vi "WPI_DashboardProcessTCPPacket.vi"(11 "data in":string) -> (1 "New Robot IP":bool, 2 "Docked":bool, 3 "Robot IP":string, 4 "Power and Errors":T1, 5 "Simulated":bool)   [LabVIEW 2025]
uses:
  <vilib>/Utility/config.llb/Read Key (String).vi
  <vilib>/Utility/config.llb/Write Key (String).vi
  <vilib>/Utility/config.llb/NI_LVConfig.lvlib
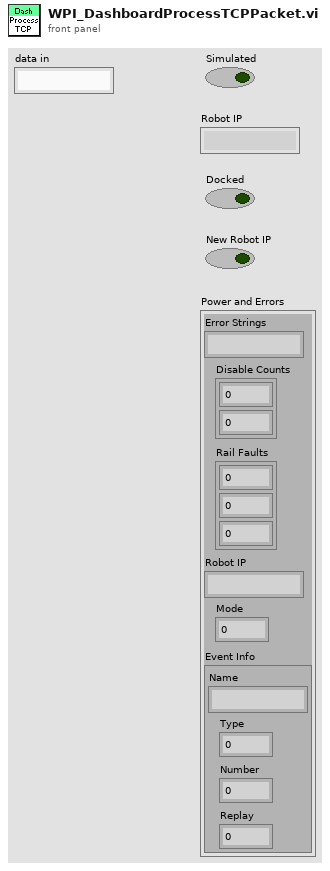
[diagram p1: front panel]
types:
  T1 = cluster{"Error Strings":string, "Disable Counts":cluster{u16, u16}, "Rail Faults":cluster{u16, u16, u16}, "Robot IP":string, "Mode":u8, "Event Info":cluster{"Name":string, "Type":u8, "Number":u16, "Replay":u8}}
  T2 = cluster{"Error Strings":string, "Disable Counts":cluster{u16, u16}, "Rail Faults":cluster{u16, u16, u16}, "Robot IP":string, "Mode":u8, "Event Info":cluster{"Name":string, "Type":u8, "Number":u16, "Replay":u8}, "New Robot IP":bool}
  T3 = typedef "NI_LVConfig.lvlib/Config Data RefNum.ctl" = refnum<k1>
  T4 = cluster{"Name":string, "Type":u8, "Number":u16, "Replay":u8}
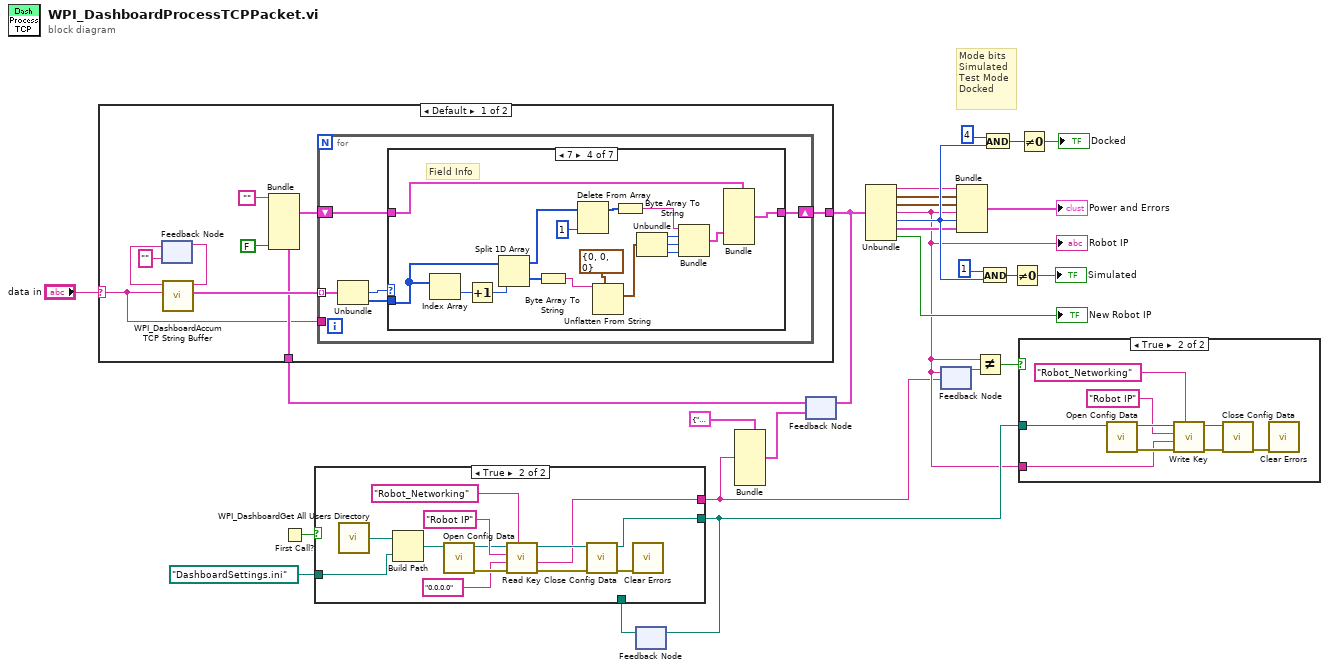
[diagram p0: block diagram]
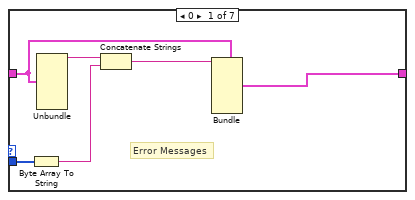
[diagram p4: hidden frame]
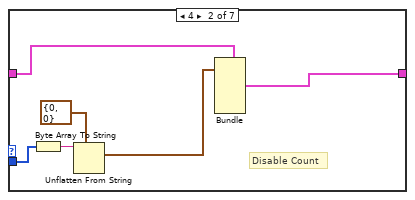
[diagram p5: hidden frame]
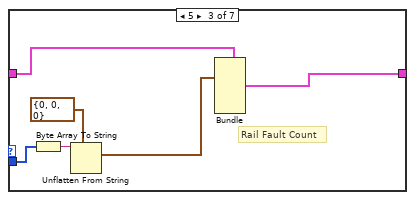
[diagram p6: hidden frame]
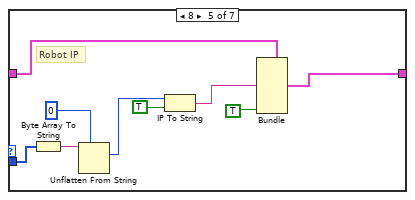
[diagram p7: hidden frame]
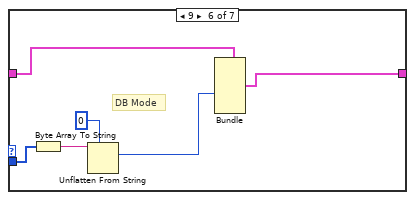
[diagram p8: hidden frame]
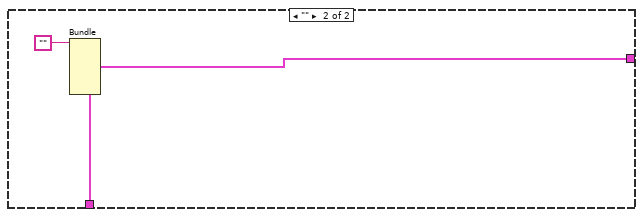
[diagram p10: hidden frame]
diagram:
  # "Mode bits\nSimulated\nTest Mode\nDocked"
  n1 = First Call?() -> (First Call?: T/F=w10:bool)
  n2 = feedback #1() -> (w3:path)  [unwired: 1 in]
  n3 = case shown="True" w10 {
    tunnel: path "DashboardSettings.ini" -> [_ w31]
    tunnel: [_ w29] -> w1
    tunnel: [w27 w28] -> w4
    tunnel: w3 -> [w27 _]
    frame False {
    }
    frame True {
      n4 = call <vilib>:"WPI_DashboardGet All Users Directory.vi"() -> ("All User Path"=w40:path)
      n5 = Build Path(base path=w40, name or relative path=w31) -> (appended path=w39:path)
      n6 = call <vilib>:"Open Config Data.vi"("configuration file path"=w39) -> ("error out"=w33:errorcluster, "refnum"=w36:T3)  [unwired: 8 in, 1 out]
      n7 = call-poly <vilib>:"Read Key.vi"("section"="Robot_Networking", "error in (no error)"=w33, "default value"="0.0.0.0", "key"="Robot IP", "refnum"=w36) -> ("error out"=w32:errorcluster, "value"=w29:string, "refnum out"=w34:T3)  [unwired: 1 in, 3 out]
      n8 = call <vilib>:"Close Config Data.vi"("error in (no error)"=w32, "refnum"=w34) -> ("error out"=w35:errorcluster, "file path"=w28:path)  [unwired: 1 in, 7 out]
      n9 = call <vilib>:"Clear Errors.vi"("error in (no error)"=w35) -> ()  [unwired: 5 in, 2 out]
    }
  }
  n10 = feedback-in #1(w4) -> ()
  n11 = Bundle(cluster=T2 {"Error Strings"="", "Disable Counts"={0, 0}, "Rail Faults"={0, 0, 0}, "Robot IP"="", "Mode"=0, "Event Info"={"Name"="", "Type"=0, "Number"=0, "Replay"=0}, "New Robot IP"=FALSE} ("Robot Info"), "Robot IP"=w1) -> (w7:T2)  [unwired: 6 in]
  n12 = feedback #2(w7) -> (w11:T2)
  n13 = case shown="Default" "data in" {
    selector: "data in" -> [w42 _]
    tunnel: [w46 w109] -> w18
    tunnel: w11 -> [w44 w108]
    frame Default {
      n14 = feedback #3("" ("string")) -> (w49:string)
      n15 = call <vilib>:"WPI_DashboardAccum TCP String Buffer.vi"("data in"=w42, "string in"=w49) -> ("Array"=w47:cluster{u16, u8, "unsigned byte array":u8[]}[], "string out"=w48:string)  [unwired: 8 in]
      n16 = feedback-in #3(w48) -> ()
      n17 = Bundle(cluster=w44, "Error Strings"="", "New Robot IP"=FALSE) -> (w43:T2)  [unwired: 5 in]
      n18 = for {
        tunnel: w47 -> [w53] mode=indexing
        shift-right: [w51] -> w46
        shift-left: w43 -> [w52]
        tunnel: w42 -> [_]
        n19 = Unbundle(w53) -> (w55:u8, "unsigned byte array"=w54:u8[])  [unwired: 1 out]
        n20 = case shown="7" w55 {
          tunnel: w54 -> [w61 w67 w73 w86 w99 w105 _]
          tunnel: w52 -> [w60 w65 w71 w90 w98 w104 w106]
          tunnel: [w56 w64 w70 w89 w97 w103 w106] -> w51
          frame 0 {
            # "Error Messages"
            n21 = Byte Array To String(unsigned byte array=w61) -> (string=w58:string)
            n22 = Unbundle(w60) -> ("Error Strings"=w59:string)  [unwired: 6 out]
            n23 = Concatenate Strings(w59, w58) -> (w57:string)
            n24 = Bundle(cluster=w60, "Error Strings"=w57) -> (w56:T2)  [unwired: 6 in]
          }
          frame 4 {
            # "Disable Count"
            n25 = Byte Array To String(unsigned byte array=w67) -> (string=w66:string)
            n26 = Unflatten From String(type=cluster{u16, u16} {0, 0}, binary string=w66) -> (value=w62:cluster{u16, u16})  [unwired: 3 in, 2 out]
            n27 = Bundle(cluster=w65, "Disable Counts"=w62) -> (w64:T2)  [unwired: 6 in]
          }
          frame 5 {
            # "Rail Fault Count"
            n28 = Byte Array To String(unsigned byte array=w73) -> (string=w72:string)
            n29 = Unflatten From String(type=cluster{u16, u16, u16} {0, 0, 0}, binary string=w72) -> (value=w68:cluster{u16, u16, u16})  [unwired: 3 in, 2 out]
            n30 = Bundle(cluster=w71, "Rail Faults"=w68) -> (w70:T2)  [unwired: 6 in]
          }
          frame 7 {
            # "Field Info"
            n31 = Index Array(array=w86) -> (element=w88:u8)  [unwired: 1 in]
            n32 = Increment(x=w88) -> (x+1=w87:u8)
            n33 = Split 1D Array(array=w86, index=w87) -> (first subarray=w82:u8[], second subarray=w84:u8[])
            n34 = Byte Array To String(unsigned byte array=w84) -> (string=w83:string)
            n35 = Delete From Array(array=w82, index=1) -> (array with subset deleted=w80:u8[])  [unwired: 1 in, 1 out]
            n36 = Unflatten From String(type=cluster{u8, u16, u8} {0, 0, 0}, binary string=w83) -> (value=w77:cluster{u8, u16, u8})  [unwired: 3 in, 2 out]
            n37 = Byte Array To String(unsigned byte array=w80) -> (string=w79:string)
            n38 = Unbundle(w77) -> (w76:u8, w75:u16, w74:u8)
            n39 = Bundle("string"=w79, w76, w75, w74) -> (w78:cluster{"string":string, u8, u16, u8})  [unwired: 1 in]
            n40 = Bundle(cluster=w90, "Event Info"=w78) -> (w89:T2)  [unwired: 6 in]
          }
          frame 8 {
            # "Robot IP"
            n41 = Byte Array To String(unsigned byte array=w99) -> (string=w96:string)
            n42 = Unflatten From String(type=u32 0, binary string=w96) -> (value=w92:u32)  [unwired: 3 in, 2 out]
            n43 = IP To String(1:TRUE ("dot notation? (F)"), 2:w92) -> (0:w91:string)
            n44 = Bundle(cluster=w98, "Robot IP"=w91, "New Robot IP"=TRUE) -> (w97:T2)  [unwired: 5 in]
          }
          frame 9 {
            # "DB Mode"
            n45 = Byte Array To String(unsigned byte array=w105) -> (string=w101:string)
            n46 = Unflatten From String(type=u8 0, binary string=w101) -> (value=w100:u8)  [unwired: 3 in, 2 out]
            n47 = Bundle(cluster=w104, "Mode"=w100) -> (w103:T2)  [unwired: 6 in]
          }
          frame Default {
          }
        }
      }
    }
    frame "" {
      n48 = Bundle(cluster=w108, "Error Strings"="") -> (w109:T2)  [unwired: 6 in]
    }
  }
  n49 = feedback-in #2(w18) -> ()
  n50 = Unbundle(w18) -> ("Error Strings"=w13:string, "Disable Counts"=w16:cluster{u16, u16}, "Rail Faults"=w15:cluster{u16, u16, u16}, "Robot IP"=w2:string, "Mode"=w25:u8, "Event Info"=w14:T4, "New Robot IP"=→"New Robot IP":bool)
  "Robot IP" <- w2
  n51 = feedback #4(w1) -> (w6:string)
  n52 = feedback-in #4(w2) -> ()
  n53 = Bundle("Error Strings"=w13, "Disable Counts"=w16, "Rail Faults"=w15, "Robot IP"=w2, "Mode"=w25, "Event Info"=w14) -> (→"Power and Errors":T1)  [unwired: 1 in]
  n54 = Not Equal?(x=w2, y=w6) -> (x != y?=w5:bool)
  n55 = And(x=1, y=w25) -> (x .and. y?=w23:i32)
  n56 = And(x=4, y=w25) -> (x .and. y?=w21:i32)
  n57 = Not Equal To 0?(x=w23) -> (x != 0?=→"Simulated":bool)
  n58 = Not Equal To 0?(x=w21) -> (x != 0?=→"Docked":bool)
  n59 = case shown="True" w5 {
    tunnel: w4 -> [_ w117]
    tunnel: w2 -> [_ w110]
    frame False {
    }
    frame True {
      n60 = call <vilib>:"Open Config Data.vi"("configuration file path"=w117) -> ("error out"=w112:errorcluster, "refnum"=w116:T3)  [unwired: 8 in, 1 out]
      n61 = call-poly <vilib>:"Write Key.vi"("section"="Robot_Networking", "error in (no error)"=w112, "value"=w110, "key"="Robot IP", "refnum"=w116) -> ("error out"=w111:errorcluster, "refnum out"=w115:T3)  [unwired: 1 in, 4 out]
      n62 = call <vilib>:"Close Config Data.vi"("error in (no error)"=w111, "refnum"=w115) -> ("error out"=w118:errorcluster)  [unwired: 1 in, 8 out]
      n63 = call <vilib>:"Clear Errors.vi"("error in (no error)"=w118) -> ()  [unwired: 5 in, 2 out]
    }
  }
